vi "test - build internal string.vi"(8 "error in (no error)":errorcluster, 11 "TestCase in":refnum<class "testcase-Basic-Function.lvclass">) -> (0 "error out":errorcluster, 3 "TestCase out":refnum<class "testcase-Basic-Function.lvclass">)   [LabVIEW 2017, in "testcase-Basic-Function.lvclass"]
uses:
  testcase-Basic-Function.lvclass
  src/user.lib/_NEVSTOP/Communicable State Machine(CSM)/_Support/Typedef/_CSM_Response Source Message.ctl
  <vilib>/addons/_JKI Toolkits/VI Tester/TestCase.llb/TestCase.lvclass
  src/user.lib/_NEVSTOP/Communicable State Machine(CSM)/Communicable State Machine.lvlib
  C:/Program Files (x86)/National Instruments/LabVIEW 2017/vi.lib/addons/_JKI Toolkits/VI Tester/TestCase.llb/TestCase.lvclass
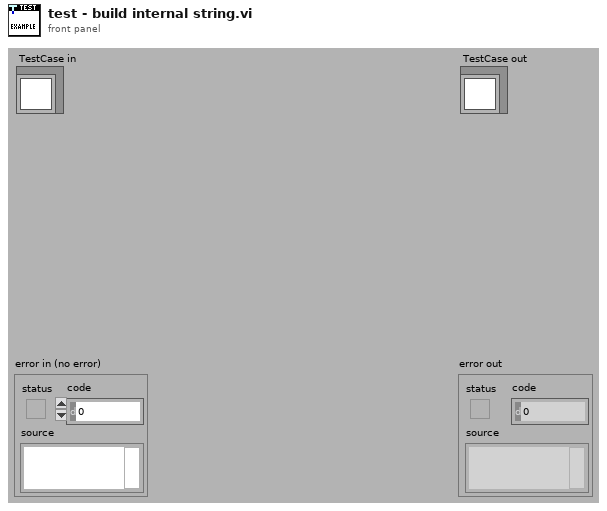
[diagram p1: front panel]
types:
  T1 = typedef "Communicable State Machine.lvlib/_CSM_Response Source Message.ctl" = cluster{"‘State":string, "’Arguments":string, "’Error":errorcluster}
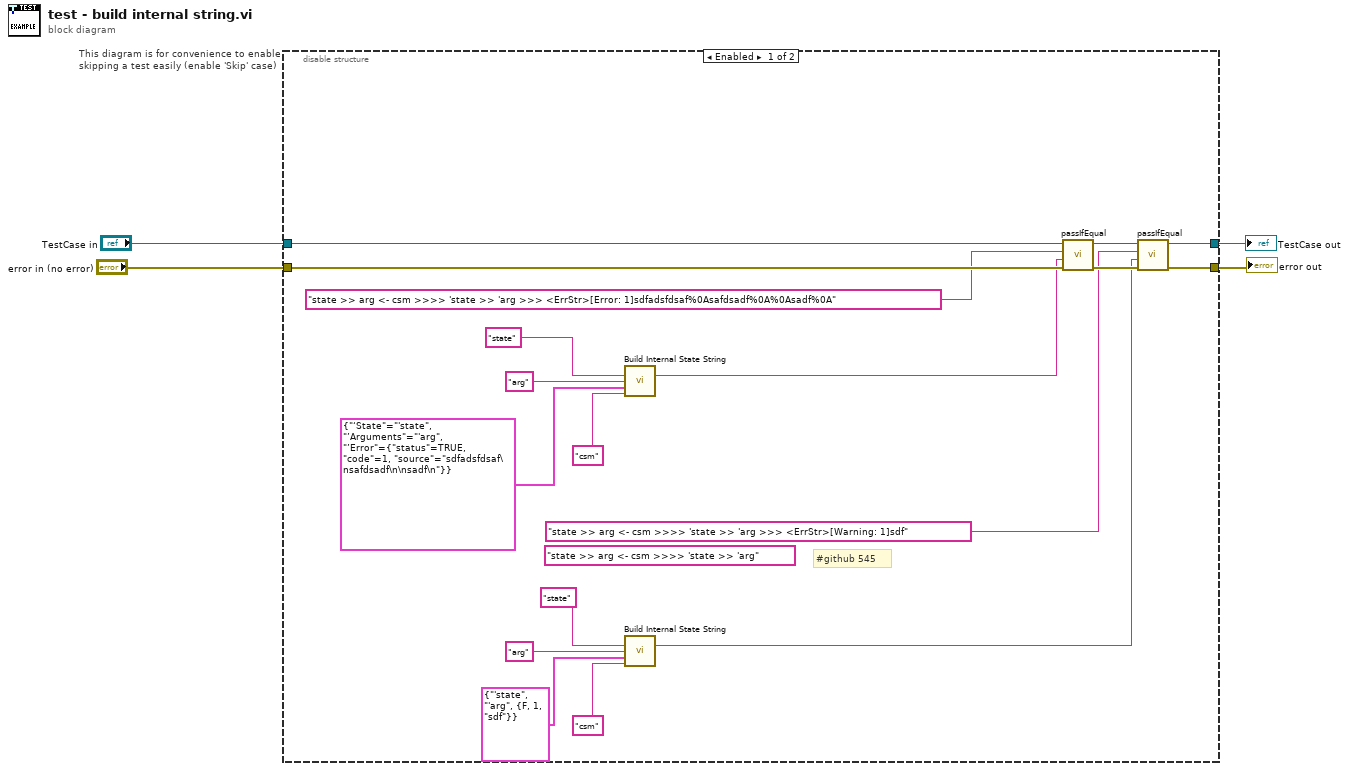
[diagram p0: block diagram]
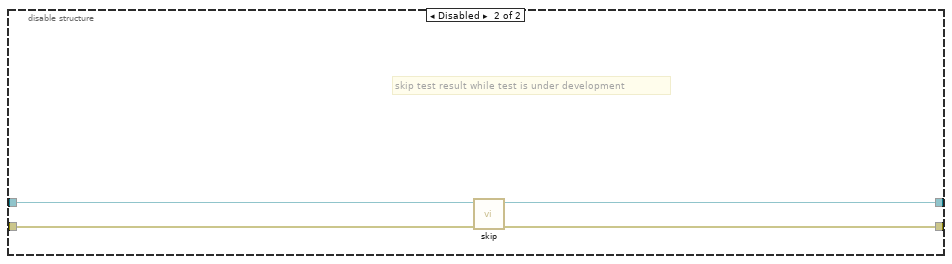
[diagram p2: hidden frame]
diagram:
  n1 = disable-structure "This diagram is for convenience to enable skipping a test easily (enable 'Skip' case)" shown="Enabled" {
    disable-tunnel: "TestCase in" -> [w22 w26]
    disable-tunnel: [w10 w24] -> w1
    disable-tunnel: [w9 w25] -> w3
    disable-tunnel: "error in (no error)" -> [w21 w23]
    frame Enabled {
      (unwired) "state >> arg <- csm >>>> 'state >> 'arg" ("State with Arguments 2")
      # "#github 545"
      n2 = call "Build Internal State String.vi"("State"="state", "Arguments (\"\")"="arg" ("Arguments (\"\")"), ">> Response Source Message >>"=T1 {"‘State"="'state", "’Arguments"="'arg", "’Error"={"status"=TRUE, "code"=1, "source"="sdfadsfdsaf\nsafdsadf\n\nsadf\n"}}, "Source (\"\")"="csm" ("Source (\"\")")) -> ("State With Arguments"=w8:string)  [unwired: 11 in]
      n3 = call "Build Internal State String.vi"("State"="state", "Arguments (\"\")"="arg" ("Arguments (\"\")"), ">> Response Source Message >>"=T1 {"‘State"="'state", "’Arguments"="'arg", "’Error"={"status"=FALSE, "code"=1, "source"="sdf"}}, "Source (\"\")"="csm" ("Source (\"\")")) -> ("State With Arguments"=w6:string)  [unwired: 11 in]
      n4 = call-dynamic "passIfEqual.vi"("error in (no error)"=w21, "y"=w8, "x"="state >> arg <- csm >>>> 'state >> 'arg >>> <ErrStr>[Error: 1]sdfadsfdsaf%0Asafdsadf%0A%0Asadf%0A" ("State with Arguments"), "TestCase in"=w22) -> ("error out"=w12:errorcluster, "TestCase out"=w11:refnum<class "testcase-Basic-Function.lvclass">)  [unwired: 6 in]
      n5 = call-dynamic "passIfEqual.vi"("error in (no error)"=w12, "y"=w6, "x"="state >> arg <- csm >>>> 'state >> 'arg >>> <ErrStr>[Warning: 1]sdf" ("State with Arguments 2"), "TestCase in"=w11) -> ("error out"=w9:errorcluster, "TestCase out"=w10:refnum<class "testcase-Basic-Function.lvclass">)  [unwired: 6 in]
    }
    frame Disabled {
      # "skip test result while test is under development"
      n6 = call <vilib>:"skip.vi"("error in (no error)"=w23, "TestCase in"=w26) -> ("error out"=w25:errorcluster, "TestCase out"=w24:refnum<class "testcase-Basic-Function.lvclass">)  [unwired: 8 in]
    }
  }
  "error out" <- w3
  "TestCase out" <- w1
